vi "下位机buffer.vi"(9 "反馈信息组":T1(array[cluster]), 10 "输入消息":T2, 11 "上传ID":u32=270 format="%x") -> (2 "输出数组":T1(array[cluster]))   [LabVIEW 2016]
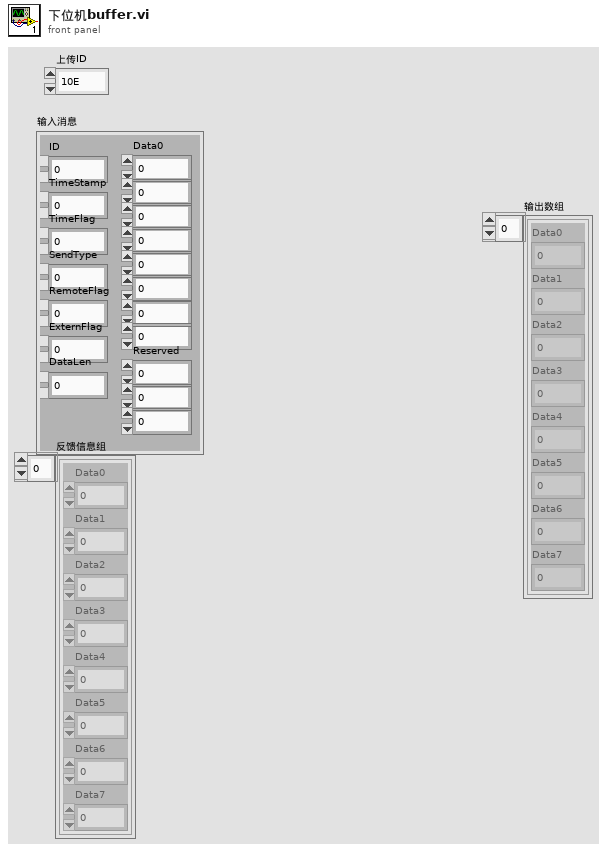
[diagram p1: front panel]
types:
  T1 = cluster{"Data0":u8, "Data1":u8, "Data2":u8, "Data3":u8, "Data4":u8, "Data5":u8, "Data6":u8, "Data7":u8}[]
  T2 = cluster{"ID":u32, "TimeStamp":u32, "TimeFlag":u8, "SendType":i8, "RemoteFlag":u8, "ExternFlag":u8, "DataLen":u8, "Data0":u64, "Data1":u64, "Data2":u64, "Data3":u64, "Data4":u64, "Data5":u64, "Data6":u64, "Data7":u64, "Reserved":u8, u8, u8}
  T3 = cluster{"Data0":u8, "Data1":u8, "Data2":u8, "Data3":u8, "Data4":u8, "Data5":u8, "Data6":u8, "Data7":u8}
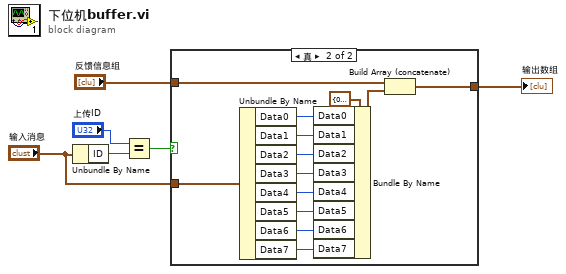
[diagram p0: block diagram]
diagram:
  n1 = Unbundle By Name("输入消息") -> ("ID"=w4:u32)
  n2 = Equal?(x="上传ID", y=w4) -> (x = y?=w6:bool)
  n3 = case shown="真" w6 {
    tunnel: "输入消息" -> [_ w20]
    tunnel: "反馈信息组" -> [w7 w9]
    tunnel: [w7 w8] -> w1
    frame False {
    }
    frame True {
      n4 = Unbundle By Name(w20) -> ("Data0"=w11:u64, "Data1"=w12:u64, "Data2"=w13:u64, "Data3"=w14:u64, "Data4"=w15:u64, "Data5"=w16:u64, "Data6"=w17:u64, "Data7"=w18:u64)
      n5 = Bundle By Name(cluster=T3 {"Data0"=0, "Data1"=0, "Data2"=0, "Data3"=0, "Data4"=0, "Data5"=0, "Data6"=0, "Data7"=0} ("簇"), "Data0"=w11, "Data1"=w12, "Data2"=w13, "Data3"=w14, "Data4"=w15, "Data5"=w16, "Data6"=w17, "Data7"=w18) -> (w10:T3)
      n6 = Build Array (concatenate)(w9, w10) -> (w8:T1)
    }
  }
  "输出数组" <- w1
